vi "HTML Report Set Font for HTML.vi"(2 "error in (no error)":errorcluster, 3 "Font Settings":T1={"Charset (-1)"=-1, "Weight (-1)"=-1, "Name"="", "Size"=" "}, 4 "Text Color (unchanged)":u32(colorbox)=16777216, 5 "HTML in":string) -> (0 "error out":errorcluster, 1 "HTML w Font Setting":string)   [LabVIEW 2015, in "NI_ReportGenerationCore.lvlib"]
doc: "This VI creates the font face and color tags for HTML documents.\n\nThe Charset (-1) and Weight (-1) don't do anything."
uses:
  <vilib>/Utility/NIReport.llb/NI_ReportGenerationCore.lvlib
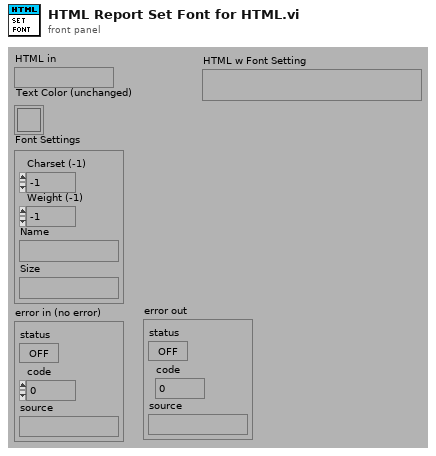
[diagram p1: front panel]
types:
  T1 = cluster{"Charset (-1)":i16, "Weight (-1)":i16, "Name":string, "Size":string}
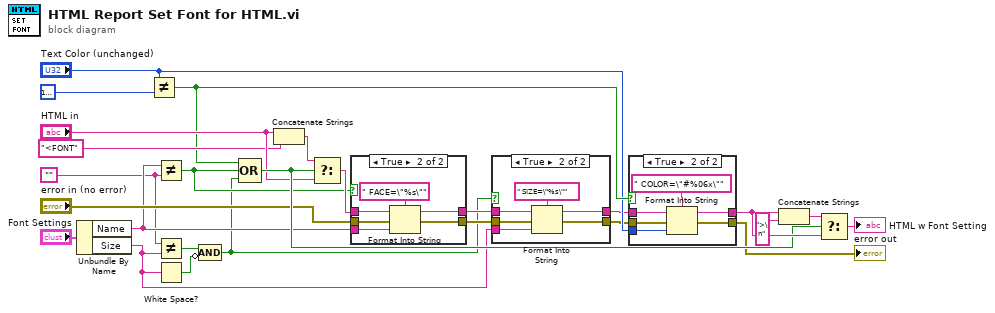
[diagram p0: block diagram]
diagram:
  w5 = "" ("Empty String Constant")
  n1 = Unbundle By Name("Font Settings") -> ("Name"=w6:string, "Size"=w3:string)
  n2 = Not Equal?(x="Text Color (unchanged)", y=u32 16777216) -> (x != y?=w16:bool)
  n3 = Not Equal?(x=w6, y=w5) -> (x != y?=w17:bool)
  n4 = Not Equal?(x=w5, y=w3) -> (x != y?=w2:bool)
  n5 = White Space?(1:w3) -> (0:w4:bool)
  n6 = Compound Arithmetic op=AND(w2, invert w4) -> (w1:bool)
  n7 = Compound Arithmetic op=OR(w16, w17, w1) -> (w22:bool)
  n8 = Concatenate Strings("HTML in", "<FONT" ("Substring")) -> (w18:string)
  n9 = Select(t=w18, s=w22, f="HTML in") -> (s? t:f=w20:string)
  n10 = case shown="True" w17 {
    tunnel: w6 -> [_ w32]
    tunnel: [w28 w34] -> w9
    tunnel: w20 -> [w28 w33]
    tunnel: "error in (no error)" -> [w27 w30]
    tunnel: [w27 w29] -> w10
    frame False {
    }
    frame True {
      n11 = Format Into String(format string=" FACE=\"%s\"" ("Format String"), initial string=w33, error in=w30, w32) -> (resulting string=w34:string, error out=w29:errorcluster)
    }
  }
  n12 = case shown="True" w1 {
    tunnel: w3 -> [_ w40]
    tunnel: [w36 w42] -> w8
    tunnel: w9 -> [w36 w41]
    tunnel: w10 -> [w35 w38]
    tunnel: [w35 w37] -> w7
    frame False {
    }
    frame True {
      n13 = Format Into String(format string=" SIZE=\"%s\"" ("Format String"), initial string=w41, error in=w38, w40) -> (resulting string=w42:string, error out=w37:errorcluster)
    }
  }
  n14 = case shown="True" w16 {
    tunnel: "Text Color (unchanged)" -> [_ w49]
    tunnel: w8 -> [w43 w46]
    tunnel: [w44 w48] -> w14
    tunnel: [w43 w47] -> w26
    tunnel: w7 -> [w44 w45]
    frame False {
    }
    frame True {
      n15 = Format Into String(format string=" COLOR=\"#%06x\"", initial string=w46, error in=w45, w49) -> (resulting string=w47:string, error out=w48:errorcluster)
    }
  }
  "error out" <- w14
  n16 = Concatenate Strings(w26, ">\n" ("Substring")) -> (w23:string)
  n17 = Select(t=w23, s=w22, f=w26) -> (s? t:f=→"HTML w Font Setting":string)
